vi "S4GUI.vi"() -> ()   [LabVIEW 2018] (continued)
                      frame #4 {
                        # "Gain"
                        n596 = Unbundle By Name(w1331) -> ("EM_GAIN"=w1330:u16)
                        n597 = Number To Decimal String(number=w1330) -> (decimal integer string=w1329:string)  [unwired: 1 in]
                      }
                      frame #5 {
                        # "Readout"
                        n598 = Unbundle By Name(w1335) -> ("EM_MODE"=w1334:u8, "READOUT_RATE"=w1333:u8)
                        n599 = case shown="0, Default" w1334 {
                          tunnel: w1333 -> [w1337 w1343]
                          tunnel: [w1336 w1342] -> w1332
                          frame 0, Default {
                            n600 = case shown="0, Default" w1337 {
                              tunnel: ["30 MHz" ("EmActive1") "20 MHz" ("EmActive1") "10 MHz" ("EmActive1") "1 MHz" ("EmActive1")] -> w1336
                              frame 0, Default {
                              }
                              frame 1 {
                              }
                              frame 2 {
                              }
                              frame 3 {
                              }
                            }
                          }
                          frame 1 {
                            n601 = case shown="1" w1343 {
                              tunnel: ["1 MHz" ("EmActive1") "0.1 MHz" ("EmActive1")] -> w1342
                              frame 0, Default {
                              }
                              frame 1 {
                              }
                            }
                          }
                        }
                      }
                    }
                  }
                }
                n602 = Unbundle By Name(w1220) -> ("INITIAL_LINE"=w1225:u16, "INITIAL_COLUMN"=w1223:u16, "FINAL_LINE"=w1226:u16, "FINAL_COLUMN"=w1224:u16, "VBIN"=w1229:u16, "HBIN"=w1285:u16, "PREAMP"=w1228:u8, "EM_GAIN"=w1227:u16, "READOUT_RATE"=w1222:u8, "SHUTTER_OPENNING_TIME"=w1284:u16, "SHUTTER_CLOSING_TIME"=w1283:u16, "VERTICAL_SHIFT_SPEED"=w1282:u8, "READ_MODE"=w1281:u8, "VERTICAL_CLOCK_VOLTAGE"=w1280:u8, "AD_CHANNEL"=w1279:u32, "SHUTTER_MODE"=w1274:u8, "SHUTTER_TTL"=w1275:u8, "TRIGGER_MODE"=w1276:u8, "FRAME_TRANSFER"=w1277:bool, "ACQUISITION_MODE"=w1278:u8, "EM_MODE"=w1221:u8)
                n603 = Not(x=w1248) -> (.not. x?=w1268:bool)
                n604 = Not(x=w1247) -> (.not. x?=w1266:bool)
                n605 = Not(x=w1246) -> (.not. x?=w1267:bool)
                n606 = Not(x=w1245) -> (.not. x?=w1265:bool)
                n607 = Not(x=w1251) -> (.not. x?=w1270:bool)
                n608 = Not(x=w1250) -> (.not. x?=w1269:bool)
                n609 = Not(x=w1249) -> (.not. x?=w1271:bool)
                n610 = property on="Image FInal Column 3" class="DigNum (strict)"("Blinking"=w1268) -> ()  [unwired: 2 in, 2 out]
                n611 = property on="Frame Transfer 3" class="Bool (strict)"("Blinking"=w1266) -> ()  [unwired: 2 in, 2 out]
                n612 = property on="Vertical Clock Voltage 3" class="Ring (strict)"("Blinking"=w1267) -> ()  [unwired: 2 in, 2 out]
                n613 = property on="A/D Channel 3" class="DigNum (strict)"("Blinking"=w1265) -> ()  [unwired: 2 in, 2 out]
                n614 = property on="Image Initial Line 3" class="DigNum (strict)"("Blinking"=w1270) -> ()  [unwired: 2 in, 2 out]
                n615 = property on="Image Initial Column 3" class="DigNum (strict)"("Blinking"=w1269) -> ()  [unwired: 2 in, 2 out]
                n616 = property on="Image Final Line 3" class="DigNum (strict)"("Blinking"=w1271) -> ()  [unwired: 2 in, 2 out]
                n617 = Not(x=w1240) -> (.not. x?=w1261:bool)
                n618 = Not(x=w1239) -> (.not. x?=w1263:bool)
                n619 = Not(x=w1238) -> (.not. x?=w1262:bool)
                n620 = Not(x=w1237) -> (.not. x?=w1264:bool)
                n621 = Not(x=w1244) -> (.not. x?=w1260:bool)
                n622 = Not(x=w1243) -> (.not. x?=w1242:bool)
                n623 = Not(x=w1241) -> (.not. x?=w1259:bool)
                n624 = property on="Shutter Openning Time 3" class="DigNum (strict)"("Blinking"=w1261) -> ()  [unwired: 2 in, 2 out]
                n625 = property on="Shutter Closing Time 3" class="DigNum (strict)"("Blinking"=w1263) -> ()  [unwired: 2 in, 2 out]
                n626 = property on="Vertical Binning 3" class="DigNum (strict)"("Blinking"=w1262) -> ()  [unwired: 2 in, 2 out]
                n627 = property on="Horizontal Binning 3" class="DigNum (strict)"("Blinking"=w1264) -> ()  [unwired: 2 in, 2 out]
                n628 = property on="CCD EM Gain 3" class="DigNum (strict)"("Blinking"=w1260) -> ()  [unwired: 2 in, 2 out]
                n629 = property on="Shutter Mode 3" class="Ring (strict)"("Blinking"=w1242) -> ()  [unwired: 2 in, 2 out]
                n630 = property on="Shutter TTL 3" class="Ring (strict)"("Blinking"=w1259) -> ()  [unwired: 2 in, 2 out]
                n631 = local read "Cameras Cluster"() -> (w1287:T6)
                n632 = Bundle By Name(cluster=w1287, "Current Configuration.Image Initial Line 3"=w1225, "Current Configuration.Image Initial Column 3"=w1223, "Current Configuration.Image Final Line 3"=w1226, "Current Configuration.Image FInal Column 3"=w1224, "Current Configuration.Vertical Binning 3"=w1229, "Current Configuration.Horizontal Binning 3"=w1285, "Current Configuration.Pre-amplification Gain 3"=w1228, "Current Configuration.CCD EM Gain 3"=w1227, "Current Configuration.Readout Rate 3"=w1222, "Current Configuration.Shutter Openning Time 3"=w1284, "Current Configuration.Shutter Closing Time 3"=w1283, "Current Configuration.Vertical Shift Speed 3"=w1282, "Current Configuration.Read Mode 3"=w1281, "Current Configuration.Vertical Clock Voltage 3"=w1280, "Current Configuration.A/D Channel 3"=w1279, "Current Configuration.Shutter Mode 3"=w1274, "Current Configuration.Shutter TTL 3"=w1275, "Current Configuration.Trigger Mode 3"=w1276, "Current Configuration.Frame Transfer 3"=w1277, "Current Configuration.Acquisition Mode 3"=w1278, "Current Configuration.CCD EM Mode 3"=w1221) -> (w1286:T6)
                n633 = Not(x=w1236) -> (.not. x?=w1252:bool)
                n634 = Not(x=w1232) -> (.not. x?=w1255:bool)
                n635 = Not(x=w1231) -> (.not. x?=w1253:bool)
                n636 = Not(x=w1230) -> (.not. x?=w1254:bool)
                n637 = Not(x=w1235) -> (.not. x?=w1257:bool)
                n638 = Not(x=w1234) -> (.not. x?=w1256:bool)
                n639 = Not(x=w1233) -> (.not. x?=w1258:bool)
                n640 = local write "RO3"(w1214) -> ()
                n641 = local write "B3"(w1216) -> ()
                n642 = local write "PA3"(w1217) -> ()
                n643 = local write "EA3"(w1218) -> ()
                n644 = local write "G3"(w1215) -> ()
                n645 = local write "SI3"(w1219) -> ()
                n646 = property on="Acquisition Mode 3" class="Ring (strict)"("Blinking"=w1252) -> ()  [unwired: 2 in, 2 out]
                n647 = property on="Readout Rate 3" class="Ring (strict)"("Blinking"=w1255) -> ()  [unwired: 2 in, 2 out]
                n648 = property on="Vertical Shift Speed 3" class="Ring (strict)"("Blinking"=w1253) -> ()  [unwired: 2 in, 2 out]
                n649 = property on="CCD EM Mode 3" class="Ring (strict)"("Blinking"=w1254) -> ()  [unwired: 2 in, 2 out]
                n650 = property on="Trigger Mode 3" class="Ring (strict)"("Blinking"=w1257) -> ()  [unwired: 2 in, 2 out]
                n651 = property on="Read Mode 3" class="Ring (strict)"("Blinking"=w1256) -> ()  [unwired: 2 in, 2 out]
                n652 = property on="Pre-amplification Gain 3" class="Ring (strict)"("Blinking"=w1258) -> ()  [unwired: 2 in, 2 out]
                n653 = local write "Cameras Cluster"(w1286) -> ()
                n654 = Compound Arithmetic op=AND(w1236, w1235, w1234, w1233, w1232, w1231, w1230, w1244, w1243, w1241, w1240, w1239, w1238, w1237, w1251, w1250, w1249, w1248, w1247, w1246, w1245) -> (→"CCD checked 3":bool)
              }
              frame #18 {
                # "Carrega coluna do Channel 4"
                # "Aba:  Eng->Camera"
                n655 = Unbundle By Name(w1421) -> ("ChannelD_CCD"=w1353:T21, "CHD_Checked Params"=w1406:T22, "ChannelD_Status.connection"=w1352:bool)
                n656 = Unbundle By Name(w1406) -> ("ACQUISITION_MODE"=w1370:bool, "TRIGGER_MODE"=w1369:bool, "READ_MODE"=w1368:bool, "PREAMP"=w1366:bool, "READOUT_RATE"=w1365:bool, "VERTICAL_SHIFT_SPEED"=w1364:bool, "EM_MODE"=w1363:bool, "EM_GAIN"=w1377:bool, "SHUTTER_MODE"=w1376:bool, "SHUTTER_TTL"=w1375:bool, "SHUTTER_OPENING_TIME"=w1374:bool, "SHUTTER_CLOSING_TIME"=w1373:bool, "VBIN"=w1372:bool, "HBIN"=w1371:bool, "INITIAL_LINE"=w1384:bool, "INITIAL_COLUMN"=w1383:bool, "FINAL_LINE"=w1382:bool, "FINAL_COLUMN"=w1381:bool, "FRAME_TRANSFER"=w1380:bool, "VERTICAL_CLOCK_VOLTAGE"=w1379:bool, "AD_CHANNEL"=w1378:bool)
                n657 = case shown="False" w1352 {
                  tunnel: w1353 -> [_ w1429]
                  tunnel: [w1422 w1428] -> w1351
                  tunnel: [w1422 w1427] -> w1350
                  tunnel: [w1422 w1426] -> w1349
                  tunnel: [w1422 w1425] -> w1348
                  tunnel: [w1422 w1424] -> w1347
                  tunnel: [w1422 w1423] -> w1346
                  frame False {
                    w1422 = ""
                  }
                  frame True {
                    n658 = stacked-sequence "Atualizacao dos indicadores inferiores do CANAL D da tela principal" {
                      tunnel: w1429 -> [w1444 w1447 w1452 w1461 w1464 w1468]
                      tunnel: [w1430 _ _ _ _ _] -> w1428
                      tunnel: [_ w1445 _ _ _ _] -> w1427
                      tunnel: [_ _ w1450 _ _ _] -> w1426
                      tunnel: [_ _ _ w1455 _ _] -> w1425
                      tunnel: [_ _ _ _ w1462 _] -> w1424
                      tunnel: [_ _ _ _ _ w1465] -> w1423
                      frame #0 {
                        # "SubImage"
                        n659 = Unbundle By Name(w1444) -> ("INITIAL_LINE"=w1442:u16, "FINAL_LINE"=w1441:u16, "INITIAL_COLUMN"=w1440:u16, "FINAL_COLUMN"=w1439:u16)
                        n660 = Number To Decimal String(number=w1442) -> (decimal integer string=w1438:string)  [unwired: 1 in]
                        n661 = Number To Decimal String(number=w1441) -> (decimal integer string=w1436:string)  [unwired: 1 in]
                        n662 = Number To Decimal String(number=w1440) -> (decimal integer string=w1434:string)  [unwired: 1 in]
                        n663 = Number To Decimal String(number=w1439) -> (decimal integer string=w1432:string)  [unwired: 1 in]
                        n664 = Concatenate Strings("[", w1438, ":", w1436, ",", w1434, ":", w1432, "]") -> (w1430:string)
                      }
                      frame #1 {
                        # "Em Active"
                        n665 = Unbundle By Name(w1447) -> ("EM_MODE"=w1446:u8)
                        n666 = case shown="0, Default" w1446 {
                          tunnel: ["Electron M." ("EmActive1") "Convent." ("EmActive1")] -> w1445
                          frame 0, Default {
                          }
                          frame 1 {
                          }
                        }
                      }
                      frame #2 {
                        # "Pre Amp"
                        n667 = Unbundle By Name(w1452) -> ("PREAMP"=w1451:u8)
                        n668 = case shown="1" w1451 {
                          tunnel: ["Gain 1" ("EmActive1") "Gain 2" ("EmActive1")] -> w1450
                          frame 0, Default {
                          }
                          frame 1 {
                          }
                        }
                      }
                      frame #3 {
                        # "Binning"
                        n669 = Unbundle By Name(w1461) -> ("VBIN"=w1460:u16, "HBIN"=w1459:u16)
                        n670 = Number To Decimal String(number=w1459) -> (decimal integer string=w1456:string)  [unwired: 1 in]
                        n671 = Number To Decimal String(number=w1460) -> (decimal integer string=w1458:string)  [unwired: 1 in]
                        n672 = Concatenate Strings(w1458, "x", w1456) -> (w1455:string)
                      }
                      frame #4 {
                        # "Gain"
                        n673 = Unbundle By Name(w1464) -> ("EM_GAIN"=w1463:u16)
                        n674 = Number To Decimal String(number=w1463) -> (decimal integer string=w1462:string)  [unwired: 1 in]
                      }
                      frame #5 {
                        # "Readout"
                        n675 = Unbundle By Name(w1468) -> ("EM_MODE"=w1467:u8, "READOUT_RATE"=w1466:u8)
                        n676 = case shown="0, Default" w1467 {
                          tunnel: w1466 -> [w1470 w1476]
                          tunnel: [w1469 w1475] -> w1465
                          frame 0, Default {
                            n677 = case shown="0, Default" w1470 {
                              tunnel: ["30 MHz" ("EmActive1") "20 MHz" ("EmActive1") "10 MHz" ("EmActive1") "1 MHz" ("EmActive1")] -> w1469
                              frame 0, Default {
                              }
                              frame 1 {
                              }
                              frame 2 {
                              }
                              frame 3 {
                              }
                            }
                          }
                          frame 1 {
                            n678 = case shown="1" w1476 {
                              tunnel: ["1 MHz" ("EmActive1") "0.1 MHz" ("EmActive1")] -> w1475
                              frame 0, Default {
                              }
                              frame 1 {
                              }
                            }
                          }
                        }
                      }
                    }
                  }
                }
                n679 = Unbundle By Name(w1353) -> ("INITIAL_LINE"=w1358:u16, "INITIAL_COLUMN"=w1356:u16, "FINAL_LINE"=w1359:u16, "FINAL_COLUMN"=w1357:u16, "VBIN"=w1362:u16, "HBIN"=w1418:u16, "PREAMP"=w1361:u8, "EM_GAIN"=w1360:u16, "READOUT_RATE"=w1355:u8, "SHUTTER_OPENNING_TIME"=w1417:u16, "SHUTTER_CLOSING_TIME"=w1416:u16, "VERTICAL_SHIFT_SPEED"=w1415:u8, "READ_MODE"=w1414:u8, "VERTICAL_CLOCK_VOLTAGE"=w1413:u8, "AD_CHANNEL"=w1412:u32, "SHUTTER_MODE"=w1407:u8, "SHUTTER_TTL"=w1408:u8, "TRIGGER_MODE"=w1409:u8, "FRAME_TRANSFER"=w1410:bool, "ACQUISITION_MODE"=w1411:u8, "EM_MODE"=w1354:u8)
                n680 = Not(x=w1381) -> (.not. x?=w1401:bool)
                n681 = Not(x=w1380) -> (.not. x?=w1399:bool)
                n682 = Not(x=w1379) -> (.not. x?=w1400:bool)
                n683 = Not(x=w1378) -> (.not. x?=w1398:bool)
                n684 = Not(x=w1384) -> (.not. x?=w1403:bool)
                n685 = Not(x=w1383) -> (.not. x?=w1402:bool)
                n686 = Not(x=w1382) -> (.not. x?=w1404:bool)
                n687 = property on="Image FInal Column 4" class="DigNum (strict)"("Blinking"=w1401) -> ()  [unwired: 2 in, 2 out]
                n688 = property on="Frame Transfer 4" class="Bool (strict)"("Blinking"=w1399) -> ()  [unwired: 2 in, 2 out]
                n689 = property on="Vertical Clock Voltage 4" class="Ring (strict)"("Blinking"=w1400) -> ()  [unwired: 2 in, 2 out]
                n690 = property on="A/D Channel 4" class="DigNum (strict)"("Blinking"=w1398) -> ()  [unwired: 2 in, 2 out]
                n691 = property on="Image Initial Line 4" class="DigNum (strict)"("Blinking"=w1403) -> ()  [unwired: 2 in, 2 out]
                n692 = property on="Image Initial Column 4" class="DigNum (strict)"("Blinking"=w1402) -> ()  [unwired: 2 in, 2 out]
                n693 = property on="Image Final Line 4" class="DigNum (strict)"("Blinking"=w1404) -> ()  [unwired: 2 in, 2 out]
                n694 = Not(x=w1374) -> (.not. x?=w1394:bool)
                n695 = Not(x=w1373) -> (.not. x?=w1396:bool)
                n696 = Not(x=w1372) -> (.not. x?=w1395:bool)
                n697 = Not(x=w1371) -> (.not. x?=w1397:bool)
                n698 = Not(x=w1377) -> (.not. x?=w1392:bool)
                n699 = Not(x=w1376) -> (.not. x?=w1393:bool)
                n700 = Not(x=w1375) -> (.not. x?=w1391:bool)
                n701 = property on="Shutter Openning Time 4" class="DigNum (strict)"("Blinking"=w1394) -> ()  [unwired: 2 in, 2 out]
                n702 = property on="Shutter Closing Time 4" class="DigNum (strict)"("Blinking"=w1396) -> ()  [unwired: 2 in, 2 out]
                n703 = property on="Vertical Binning 4" class="DigNum (strict)"("Blinking"=w1395) -> ()  [unwired: 2 in, 2 out]
                n704 = property on="Horizontal Binning 4" class="DigNum (strict)"("Blinking"=w1397) -> ()  [unwired: 2 in, 2 out]
                n705 = property on="CCD EM Gain 4" class="DigNum (strict)"("Blinking"=w1392) -> ()  [unwired: 2 in, 2 out]
                n706 = property on="Shutter Mode 4" class="Ring (strict)"("Blinking"=w1393) -> ()  [unwired: 2 in, 2 out]
                n707 = property on="Shutter TTL 4" class="Ring (strict)"("Blinking"=w1391) -> ()  [unwired: 2 in, 2 out]
                n708 = local read "Cameras Cluster"() -> (w1420:T6)
                n709 = Bundle By Name(cluster=w1420, "Current Configuration.Image Initial Line 4"=w1358, "Current Configuration.Image Initial Column 4"=w1356, "Current Configuration.Image Final Line 4"=w1359, "Current Configuration.Image FInal Column 4"=w1357, "Current Configuration.Vertical Binning 4"=w1362, "Current Configuration.Horizontal Binning 4"=w1418, "Current Configuration.Pre-amplification Gain 4"=w1361, "Current Configuration.CCD EM Gain 4"=w1360, "Current Configuration.Readout Rate 4"=w1355, "Current Configuration.Shutter Openning Time 4"=w1417, "Current Configuration.Shutter Closing Time 4"=w1416, "Current Configuration.Vertical Shift Speed 4"=w1415, "Current Configuration.Read Mode 4"=w1414, "Current Configuration.Vertical Clock Voltage 4"=w1413, "Current Configuration.A/D Channel 4"=w1412, "Current Configuration.Shutter Mode 4"=w1407, "Current Configuration.Shutter TTL 4"=w1408, "Current Configuration.Trigger Mode 4"=w1409, "Current Configuration.Frame Transfer 4"=w1410, "Current Configuration.Acquisition Mode 4"=w1411, "Current Configuration.CCD EM Mode 4"=w1354) -> (w1419:T6)
                n710 = local write "SI4"(w1351) -> ()
                n711 = local write "RO4"(w1346) -> ()
                n712 = local write "PA4"(w1349) -> ()
                n713 = local write "EA4"(w1350) -> ()
                n714 = local write "G4"(w1347) -> ()
                n715 = local write "B4"(w1348) -> ()
                n716 = Not(x=w1370) -> (.not. x?=w1385:bool)
                n717 = Not(x=w1365) -> (.not. x?=w1388:bool)
                n718 = Not(x=w1364) -> (.not. x?=w1386:bool)
                n719 = Not(x=w1363) -> (.not. x?=w1387:bool)
                n720 = Not(x=w1369) -> (.not. x?=w1389:bool)
                n721 = Not(x=w1368) -> (.not. x?=w1367:bool)
                n722 = Not(x=w1366) -> (.not. x?=w1390:bool)
                n723 = property on="Acquisition Mode 4" class="Ring (strict)"("Blinking"=w1385) -> ()  [unwired: 2 in, 2 out]
                n724 = property on="Readout Rate 4" class="Ring (strict)"("Blinking"=w1388) -> ()  [unwired: 2 in, 2 out]
                n725 = property on="Vertical Shift Speed 4" class="Ring (strict)"("Blinking"=w1386) -> ()  [unwired: 2 in, 2 out]
                n726 = property on="CCD EM Mode 4" class="Ring (strict)"("Blinking"=w1387) -> ()  [unwired: 2 in, 2 out]
                n727 = property on="Trigger Mode 4" class="Ring (strict)"("Blinking"=w1389) -> ()  [unwired: 2 in, 2 out]
                n728 = property on="Read Mode 4" class="Ring (strict)"("Blinking"=w1367) -> ()  [unwired: 2 in, 2 out]
                n729 = property on="Pre-amplification Gain 4" class="Ring (strict)"("Blinking"=w1390) -> ()  [unwired: 2 in, 2 out]
                n730 = local write "Cameras Cluster"(w1419) -> ()
                n731 = Compound Arithmetic op=AND(w1370, w1369, w1368, w1366, w1365, w1364, w1363, w1377, w1376, w1375, w1374, w1373, w1372, w1371, w1384, w1383, w1382, w1381, w1380, w1379, w1378) -> (→"CCD checked 4":bool)
              }
            }
            n732 = stacked-sequence {
              tunnel: w172 -> [w186 w190 w198 w205 w219]
              tunnel: w171 -> [w185 w189 w197 w204 w218]
              tunnel: [_ _ _ _ w210] -> w163
              tunnel: [_ _ _ _ w211] -> w162
              frame #0 {
                n733 = call-dynamic "Read AcquisitionA.vi"("error in (no error)"=w185, "S4ACS_GUI in"=w186) -> ("error out"=w182:errorcluster, "Acquisition.lvclass"=w184:refnum<class "Acquisition.lvclass">)  [unwired: 7 in, 1 out]
                n734 = call-dynamic "Read Channel.vi"("error in (no error)"=w182, "Acquisition in"=w184) -> ("error out"=w181:errorcluster, "Channel.lvclass"=w183:refnum<class "Channel.lvclass">)  [unwired: 7 in, 1 out]
                n735 = call-dynamic "Read CyclesDone.vi"("error in (no error)"=w181, "Channel in"=w183) -> ("error out"=→"error out 6":errorcluster, "CyclesDone"=→"Cycles Done ch1":u32)  [unwired: 7 in, 1 out]
              }
              frame #1 {
                n736 = call "Read AcquisitionB.vi"("error in (no error)"=w189, "S4ACS_GUI in"=w190) -> ("error out"=w192:errorcluster, "Acquisition.lvclass"=w193:refnum<class "Acquisition.lvclass">)  [unwired: 7 in, 1 out]
                n737 = call-dynamic "Read Channel.vi"("error in (no error)"=w192, "Acquisition in"=w193) -> ("error out"=w191:errorcluster, "Channel.lvclass"=w194:refnum<class "Channel.lvclass">)  [unwired: 7 in, 1 out]
                n738 = call-dynamic "Read CyclesDone.vi"("error in (no error)"=w191, "Channel in"=w194) -> ("error out"=→"error out 4":errorcluster, "CyclesDone"=→"Cycles Done ch2":u32)  [unwired: 7 in, 1 out]
              }
              frame #2 {
                n739 = call-dynamic "Read AcquisitionC.vi"("error in (no error)"=w197, "S4ACS_GUI in"=w198) -> ("error out"=w200:errorcluster, "Acquisition.lvclass"=w201:refnum<class "Acquisition.lvclass">)  [unwired: 7 in, 1 out]
                n740 = call-dynamic "Read Channel.vi"("error in (no error)"=w200, "Acquisition in"=w201) -> ("error out"=w199:errorcluster, "Channel.lvclass"=w202:refnum<class "Channel.lvclass">)  [unwired: 7 in, 1 out]
                n741 = call-dynamic "Read CyclesDone.vi"("error in (no error)"=w199, "Channel in"=w202) -> ("error out"=→"error out 5":errorcluster, "CyclesDone"=→"Cycles Done ch3":u32)  [unwired: 7 in, 1 out]
              }
              frame #3 {
                n742 = call-dynamic "Read AcquisitionD.vi"("error in (no error)"=w204, "S4ACS_GUI in"=w205) -> ("error out"=w207:errorcluster, "Acquisition.lvclass"=w208:refnum<class "Acquisition.lvclass">)  [unwired: 7 in, 1 out]
                n743 = call-dynamic "Read Channel.vi"("error in (no error)"=w207, "Acquisition in"=w208) -> ("error out"=w206:errorcluster, "Channel.lvclass"=w209:refnum<class "Channel.lvclass">)  [unwired: 7 in, 1 out]
                n744 = call-dynamic "Read CyclesDone.vi"("error in (no error)"=w206, "Channel in"=w209) -> ("CyclesDone"=→"Cycles Done ch4":u32)  [unwired: 7 in, 2 out]
              }
              frame #4 {
                (unwired) cluster{"AG status":bool, "rotator":dbl} {"AG status"=FALSE, "rotator"=0.0} ("element")
                n745 = call-dynamic "Read guider queue.vi"("error in (no error)"=w218, "S4GUI in"=w219) -> ("error out"=w213:errorcluster, "guider queue"=w217:refnum<queue>, "S4GUI out"=w212:refnum<class "S4GUI.lvclass">)  [unwired: 7 in]
                n746 = Get Queue Status(queue=w217, error in (no error)=w213) -> (queue out=w215:refnum<queue>, error out=w214:errorcluster, # elements in queue=w216:i32)  [unwired: 1 in, 5 out]
                n747 = case shown="Default" w216 {
                  tunnel: w215 -> [_ w232]
                  tunnel: w214 -> [w220 w231]
                  tunnel: w212 -> [w221 w226]
                  tunnel: [w220 w224] -> w211
                  tunnel: [w221 w225] -> w210
                  frame 0 {
                  }
                  frame Default {
                    n748 = Dequeue Element(queue=w232, error in (no error)=w231) -> (queue out=w229:refnum<queue>, element=w228:cluster{"AG status":bool, "rotator":dbl}, error out=w230:errorcluster)  [unwired: 1 in, 1 out]
                    n749 = Unbundle By Name(w228) -> ("AG status"=→"GUIDER":bool, "rotator"=w222:dbl)
                    "rotator" <- w222
                    n750 = Flush Queue(queue=w229, error in (no error)=w230) -> (error out=w223:errorcluster)  [unwired: 2 out]
                    n751 = call-dynamic "Write rotator.vi"("error in (no error)"=w223, "rotator"=w222, "S4GUI in"=w226) -> ("error out"=w224:errorcluster, "S4GUI out"=w225:refnum<class "S4GUI.lvclass">)  [unwired: 7 in]
                  }
                }
              }
            }
            n752 = call-dynamic "Read Obs_state.vi"("error in (no error)"=w162, "S4ACS_GUI in"=w163) -> ("error out"=w158:errorcluster, "Obs_state"=w159:u32, "S4ACS_GUI out"=w157:refnum<class "S4GUI.lvclass">)  [unwired: 7 in]
            n753 = In Range and Coerce(upper limit=u32 226, x=w159, lower limit=u32 220 ("upper limit")) -> (In Range?=w155:bool)  [unwired: 1 out]
            n754 = Select(t="STOP", s=w155, f="INIT") -> (s? t:f=w154:string)
            n755 = property on="Init mode" class="Bool"(error in=w158, "Blinking"=w155, "Caption.Visible"=w155, "BoolText.Text"=w154) -> (error out=w156:errorcluster)  [unwired: 1 in, 1 out]
            n756 = call-dynamic "Read cyclesDone.vi"("error in (no error)"=w156, "S4GUI in"=w157) -> ("error out"=w174:errorcluster, "cyclesDone"=→"#Cycles Done":u32, "S4GUI out"=w173:refnum<class "S4GUI.lvclass">)  [unwired: 7 in]
            n757 = call "Read Instrument.lvclass.vi"("error in (no error)"=w174, "S4ACS_GUI in"=w173) -> ("error out"=w168:errorcluster, "Instrument.lvclass"=w165:refnum<class "Instrument.lvclass">, "S4ACS_GUI out"=w170:refnum<class "S4GUI.lvclass">)  [unwired: 7 in]
            n758 = call-dynamic "Write mode.vi"("error in (no error)"=w168, "mode"=w150, "Instrument in"=w165) -> ("error out"=w167:errorcluster, "Instrument out"=w164:refnum<class "Instrument.lvclass">)  [unwired: 7 in]
            n759 = call "Write Instrument.lvclass.vi"("error in (no error)"=w167, "Instrument.lvclass"=w164, "S4ACS_GUI in"=w170) -> ("error out"=w166:errorcluster, "S4ACS_GUI out"=w169:refnum<class "S4GUI.lvclass">)  [unwired: 7 in]
          }
        }
        n760 = Or(x="stop", y="stop 2") -> (x .or. y?=w133:bool)
      }
      event "Set from Input ch1": Value Change {
        # "ACS"
        # "GUI"
        # "EM_MODE = E.M."
        # "Readou Rate:\n30         0\n20         1     \n10         2\n1           3"
        # "EM_MODE = Conv"
        # "Readou Rate:\n1         0\n0.1      1"
        # "Readou Rate:\n1         0\n0.1      1     \n10       2\n20       3\n30       4"
        n761 = event-data() -> ()  [unwired: 1 in, 6 out]
        n762 = local read "Input Cluster"() -> (w1489:T5)
        n763 = Unbundle By Name(w1489) -> ("Parameters"=w1488:T23)
        n764 = Unbundle By Name(w1488) -> ("Image \nInitial Line"=w1517:u16, "Image\nInitial Column"=w1516:u16, "Image\nFinal Line"=w1515:u16, "Image\nFInal Column"=w1514:u16, "Vertical\nBinning"=w1513:u16, "Horizontal\nBinning"=w1512:u16, "Pre-amplification\nGain"=w1511:u8, "CCD\nEM Gain"=w1510:u16, "Readout\nRate"=w1509:u8, "Shutter\nOpenning Time"=w1508:i32, "Shutter\nClosing Time"=w1507:i32, "Vertical\nShift Speed"=w1506:u8, "Read\nMode"=w1505:u8, "Vertical\nClock Voltage"=w1504:u8, "A/D \nChannel"=w1503:u32, "Shutter\nMode"=w1502:u16, "Shutter\nTTL"=w1501:u16, "Trigger\nMode"=w1500:u16, "Frame\nTransfer"=w1499:bool, "Acquisition\nMode"=w1498:u8, "CCD \nEM Mode"=w1497:u8)
        n765 = call-dynamic "Read AcquisitionA.vi"("error in (no error)"=w1480, "S4ACS_GUI in"=w1481) -> ("error out"=w1540:errorcluster, "Acquisition.lvclass"=w1544:refnum<class "Acquisition.lvclass">, "S4ACS_GUI out"=w1545:refnum<class "S4GUI.lvclass">)  [unwired: 7 in]
        n766 = call-dynamic "Read Channel.vi"("error in (no error)"=w1540, "Acquisition in"=w1544) -> ("error out"=w1539:errorcluster, "Channel.lvclass"=w1542:refnum<class "Channel.lvclass">, "Acquisition out"=w1543:refnum<class "Acquisition.lvclass">)  [unwired: 7 in]
        n767 = call-dynamic "Read Interface.vi"("error in (no error)"=w1539, "Channel in"=w1542) -> ("error out"=w1521:errorcluster, "Interface.lvclass"=w1522:refnum<class "Interface.lvclass">, "Channel out"=w1541:refnum<class "Channel.lvclass">)  [unwired: 7 in]
        n768 = call-dynamic "Get CCD_Config.vi"("error in (no error)"=w1521, "Interface in"=w1522) -> ("error out"=w1518:errorcluster, "output cluster"=w1520:T24, "Interface out"=w1519:refnum<class "Interface.lvclass">)  [unwired: 7 in]
        n769 = Bundle By Name(cluster=w1520, "INITIAL_LINE"=w1517, "INITIAL_COLUMN"=w1516, "FINAL_LINE"=w1515, "FINAL_COLUMN"=w1514, "VBIN"=w1513, "HBIN"=w1512, "PREAMP"=w1511, "EM_GAIN"=w1510, "READOUT_RATE"=w1509, "SHUTTER_OPENING_TIME"=w1508, "SHUTTER_CLOSING_TIME"=w1507, "VERTICAL_SHIFT_SPEED"=w1506, "READ_MODE"=w1505, "VERTICAL_CLOCK_VOLTAGE"=w1504, "AD_CHANNEL"=w1503, "SHUTTER_MODE"=w1502, "SHUTTER_TTL"=w1501, "TRIGGER_MODE"=w1500, "FRAME_TRANSFER"=w1499, "ACQUISITION_MODE"=w1498, "EM_MODE"=w1497) -> (w1487:T24)
        n770 = call-dynamic "Set CCD_Config.vi"("error in (no error)"=w1518, "input cluster"=w1487, "Interface in"=w1519) -> ("error out"=w1525:errorcluster, "Interface out"=w1526:refnum<class "Interface.lvclass">)  [unwired: 7 in]
        n771 = Flatten To String(anything=w1487, error in (no error)=w1525) -> (data string=w1528:string, error out=w1527:errorcluster)  [unwired: 2 in, 1 out]
        n772 = call "Write flatted cluster.vi"("error in (no error)"=w1527, "flatted cluster"=w1528, "Interface in"=w1526) -> ("error out"=w1524:errorcluster, "Interface out"=w1523:refnum<class "Interface.lvclass">)  [unwired: 7 in]
        n773 = call-dynamic "Write Interface.vi"("error in (no error)"=w1524, "Interface.lvclass"=w1523, "Channel in"=w1541) -> ("error out"=w1492:errorcluster, "Channel out"=w1495:refnum<class "Channel.lvclass">)  [unwired: 7 in]
        n774 = call "Write section_name.vi"("error in (no error)"=w1492, "section_name"="CCD_ACS1", "Channel in"=w1495) -> ("error out"=w1491:errorcluster, "Channel out"=w1494:refnum<class "Channel.lvclass">)  [unwired: 7 in]
        n775 = call-dynamic "save config.vi"("error in (no error)"=w1491, "file config"="lastsaved.cfg", "Channel in"=w1494) -> ("error out"=w1490:errorcluster, "Channel out"=w1493:refnum<class "Channel.lvclass">)  [unwired: 7 in]
        n776 = call-dynamic "Read State Machine.vi"("error in (no error)"=w1490, "Device in"=w1493) -> ("error out"=w1535:errorcluster, "State Machine.lvclass"=w1537:refnum<class "State Machine.lvclass">, "Device out"=w1538:refnum<class "Channel.lvclass">)  [unwired: 7 in]
        n777 = call-dynamic "Write State.vi"("error in (no error)"=w1535, "State"=60, "State Machine in"=w1537) -> ("error out"=w1534:errorcluster, "State Machine out"=w1536:refnum<class "State Machine.lvclass">)  [unwired: 7 in]
        n778 = call-dynamic "Write State Machine.vi"("error in (no error)"=w1534, "State Machine.lvclass"=w1536, "Device in"=w1538) -> ("error out"=w1531:errorcluster, "Device out"=w1532:refnum<class "Channel.lvclass">)  [unwired: 7 in]
        n779 = call-dynamic "Write Channel.vi"("error in (no error)"=w1531, "Channel.lvclass"=w1532, "Acquisition in"=w1543) -> ("error out"=w1530:errorcluster, "Acquisition out"=w1529:refnum<class "Acquisition.lvclass">)  [unwired: 7 in]
        n780 = call-dynamic "Write AcquisitionA.vi"("error in (no error)"=w1530, "Acquisition.lvclass"=w1529, "S4ACS_GUI in"=w1545) -> ("error out"=w1482:errorcluster, "S4ACS_GUI out"=w1483:refnum<class "S4GUI.lvclass">)  [unwired: 7 in]
        n781 = call "Write cfg file.vi"("error in (no error)"=w1482, "cfg file"="lastsaved.cfg", "S4ACS_GUI in"=w1483) -> ("error out"=w1485:errorcluster, "S4ACS_GUI out"=w1486:refnum<class "S4GUI.lvclass">)  [unwired: 7 in]
      }
      event "Input Cluster.Parameters.CCD \nEM Mode": Value Change {
        n782 = event-data() -> ()  [unwired: 1 in, 6 out]
        n783 = local read "Input Cluster"() -> (w1560:T5)
        n784 = Unbundle By Name(w1560) -> ("Parameters"=w1561:T23)
        n785 = Unbundle By Name(w1561) -> ("Readout\nRate"=→"Readout\nRate":u8, "CCD \nEM Mode"=w1555:u8)
        n786 = case shown="1" w1555 {
          tunnel: [string[] ["30 MHz", "20 MHz", "10 MHz", "1 MHz"] ("Strings []") string[] ["1 MHz", "0.1 MHz"] ("Strings []")] -> w1554
          tunnel: [u8 3 u8 0] -> w1553
          frame 0, Default {
          }
          frame 1 {
          }
        }
        n787 = local read "Cameras Cluster"() -> (w1548:T6)
        n788 = Unbundle By Name(w1548) -> ("Current Configuration"=w1549:T25)
        n789 = flat-sequence {
          tunnel: w1553 -> [w1563]
          tunnel: w1554 -> [w1562]
          tunnel: w1555 -> [w1564]
          tunnel: [w1564] -> w1552
          tunnel: [w1563] -> w1550
          tunnel: w1561 -> [w1570]
          tunnel: [w1569] -> w1559
          tunnel: w1552 -> [w1565]
          tunnel: w1550 -> [w1566]
          tunnel: w1549 -> [w1568]
          tunnel: [w1567] -> w1547
          frame #0 {
            n790 = property on="Readout\nRate" class="Ring (strict)"("Strings []"=w1562) -> ()  [unwired: 2 in, 2 out]
            n791 = property on="Readout Rate" class="Ring (strict)"("Strings []"=w1562) -> ()  [unwired: 2 in, 2 out]
            n792 = property on="Readout Rate 4" class="Ring (strict)"("Strings []"=w1562) -> ()  [unwired: 2 in, 2 out]
            n793 = property on="Readout Rate 2" class="Ring (strict)"("Strings []"=w1562) -> ()  [unwired: 2 in, 2 out]
            n794 = property on="Readout Rate 3" class="Ring (strict)"("Strings []"=w1562) -> ()  [unwired: 2 in, 2 out]
          }
          frame #1 {
            n795 = Bundle By Name(cluster=w1568, "Readout Rate"=w1566, "Read Mode"=w1565) -> (w1567:T25)
            n796 = Bundle By Name(cluster=w1570, "Readout\nRate"=w1566, "CCD \nEM Mode"=w1565) -> (w1569:T23)
          }
        }
        n797 = Bundle By Name(cluster=w1560, "Parameters"=w1559) -> (w1558:T5)
        n798 = Bundle By Name(cluster=w1548, "Current Configuration"=w1547) -> (w1546:T6)
        n799 = local write "Input Cluster"(w1558) -> ()
        n800 = local write "Cameras Cluster"(w1546) -> ()
      }
      event "Set from Input ch2": Value Change {
        n801 = event-data() -> ()  [unwired: 1 in, 6 out]
        n802 = local read "Input Cluster"() -> (w1583:T5)
        n803 = Unbundle By Name(w1583) -> ("Parameters"=w1582:T23)
        n804 = Unbundle By Name(w1582) -> ("Image \nInitial Line"=w1611:u16, "Image\nInitial Column"=w1610:u16, "Image\nFinal Line"=w1609:u16, "Image\nFInal Column"=w1608:u16, "Vertical\nBinning"=w1607:u16, "Horizontal\nBinning"=w1606:u16, "Pre-amplification\nGain"=w1605:u8, "CCD\nEM Gain"=w1604:u16, "Readout\nRate"=w1603:u8, "Shutter\nOpenning Time"=w1602:i32, "Shutter\nClosing Time"=w1601:i32, "Vertical\nShift Speed"=w1600:u8, "Read\nMode"=w1599:u8, "Vertical\nClock Voltage"=w1598:u8, "A/D \nChannel"=w1597:u32, "Shutter\nMode"=w1596:u16, "Shutter\nTTL"=w1595:u16, "Trigger\nMode"=w1594:u16, "Frame\nTransfer"=w1593:bool, "Acquisition\nMode"=w1592:u8, "CCD \nEM Mode"=w1591:u8)
        n805 = call "Read AcquisitionB.vi"("error in (no error)"=w1640, "S4ACS_GUI in"=w1641) -> ("error out"=w1634:errorcluster, "Acquisition.lvclass"=w1638:refnum<class "Acquisition.lvclass">, "S4ACS_GUI out"=w1639:refnum<class "S4GUI.lvclass">)  [unwired: 7 in]
        n806 = call-dynamic "Read Channel.vi"("error in (no error)"=w1634, "Acquisition in"=w1638) -> ("error out"=w1633:errorcluster, "Channel.lvclass"=w1636:refnum<class "Channel.lvclass">, "Acquisition out"=w1637:refnum<class "Acquisition.lvclass">)  [unwired: 7 in]
        n807 = call-dynamic "Read Interface.vi"("error in (no error)"=w1633, "Channel in"=w1636) -> ("error out"=w1615:errorcluster, "Interface.lvclass"=w1616:refnum<class "Interface.lvclass">, "Channel out"=w1635:refnum<class "Channel.lvclass">)  [unwired: 7 in]
        n808 = call-dynamic "Get CCD_Config.vi"("error in (no error)"=w1615, "Interface in"=w1616) -> ("error out"=w1612:errorcluster, "output cluster"=w1614:T24, "Interface out"=w1613:refnum<class "Interface.lvclass">)  [unwired: 7 in]
        n809 = Bundle By Name(cluster=w1614, "INITIAL_LINE"=w1611, "INITIAL_COLUMN"=w1610, "FINAL_LINE"=w1609, "FINAL_COLUMN"=w1608, "VBIN"=w1607, "HBIN"=w1606, "PREAMP"=w1605, "EM_GAIN"=w1604, "READOUT_RATE"=w1603, "SHUTTER_OPENING_TIME"=w1602, "SHUTTER_CLOSING_TIME"=w1601, "VERTICAL_SHIFT_SPEED"=w1600, "READ_MODE"=w1599, "VERTICAL_CLOCK_VOLTAGE"=w1598, "AD_CHANNEL"=w1597, "SHUTTER_MODE"=w1596, "SHUTTER_TTL"=w1595, "TRIGGER_MODE"=w1594, "FRAME_TRANSFER"=w1593, "ACQUISITION_MODE"=w1592, "EM_MODE"=w1591) -> (w1581:T24)
        n810 = call-dynamic "Set CCD_Config.vi"("error in (no error)"=w1612, "input cluster"=w1581, "Interface in"=w1613) -> ("error out"=w1619:errorcluster, "Interface out"=w1620:refnum<class "Interface.lvclass">)  [unwired: 7 in]
        n811 = Flatten To String(anything=w1581, error in (no error)=w1619) -> (data string=w1622:string, error out=w1621:errorcluster)  [unwired: 2 in, 1 out]
        n812 = call "Write flatted cluster.vi"("error in (no error)"=w1621, "flatted cluster"=w1622, "Interface in"=w1620) -> ("error out"=w1618:errorcluster, "Interface out"=w1617:refnum<class "Interface.lvclass">)  [unwired: 7 in]
        n813 = call-dynamic "Write Interface.vi"("error in (no error)"=w1618, "Interface.lvclass"=w1617, "Channel in"=w1635) -> ("error out"=w1586:errorcluster, "Channel out"=w1589:refnum<class "Channel.lvclass">)  [unwired: 7 in]
        n814 = call "Write section_name.vi"("error in (no error)"=w1586, "section_name"="CCD_ACS2", "Channel in"=w1589) -> ("error out"=w1585:errorcluster, "Channel out"=w1588:refnum<class "Channel.lvclass">)  [unwired: 7 in]
        n815 = call-dynamic "save config.vi"("error in (no error)"=w1585, "file config"="lastsaved.cfg", "Channel in"=w1588) -> ("error out"=w1584:errorcluster, "Channel out"=w1587:refnum<class "Channel.lvclass">)  [unwired: 7 in]
        n816 = call-dynamic "Read State Machine.vi"("error in (no error)"=w1584, "Device in"=w1587) -> ("error out"=w1629:errorcluster, "State Machine.lvclass"=w1631:refnum<class "State Machine.lvclass">, "Device out"=w1632:refnum<class "Channel.lvclass">)  [unwired: 7 in]
        n817 = call-dynamic "Write State.vi"("error in (no error)"=w1629, "State"=60, "State Machine in"=w1631) -> ("error out"=w1628:errorcluster, "State Machine out"=w1630:refnum<class "State Machine.lvclass">)  [unwired: 7 in]
        n818 = call-dynamic "Write State Machine.vi"("error in (no error)"=w1628, "State Machine.lvclass"=w1630, "Device in"=w1632) -> ("error out"=w1625:errorcluster, "Device out"=w1626:refnum<class "Channel.lvclass">)  [unwired: 7 in]
        n819 = call-dynamic "Write Channel.vi"("error in (no error)"=w1625, "Channel.lvclass"=w1626, "Acquisition in"=w1637) -> ("error out"=w1624:errorcluster, "Acquisition out"=w1623:refnum<class "Acquisition.lvclass">)  [unwired: 7 in]
        n820 = call "Write AcquisitionB.vi"("error in (no error)"=w1624, "Acquisition.lvclass"=w1623, "S4ACS_GUI in"=w1639) -> ("error out"=w1575:errorcluster, "S4ACS_GUI out"=w1576:refnum<class "S4GUI.lvclass">)  [unwired: 7 in]
        n821 = call "Write cfg file.vi"("error in (no error)"=w1575, "cfg file"="lastsaved.cfg", "S4ACS_GUI in"=w1576) -> ("error out"=w1578:errorcluster, "S4ACS_GUI out"=w1579:refnum<class "S4GUI.lvclass">)  [unwired: 7 in]
      }
      event "Set from Input ch3": Value Change {
        n822 = event-data() -> ()  [unwired: 1 in, 6 out]
        n823 = local read "Input Cluster"() -> (w1650:T5)
        n824 = Unbundle By Name(w1650) -> ("Parameters"=w1649:T23)
        n825 = Unbundle By Name(w1649) -> ("Image \nInitial Line"=w1678:u16, "Image\nInitial Column"=w1677:u16, "Image\nFinal Line"=w1676:u16, "Image\nFInal Column"=w1675:u16, "Vertical\nBinning"=w1674:u16, "Horizontal\nBinning"=w1673:u16, "Pre-amplification\nGain"=w1672:u8, "CCD\nEM Gain"=w1671:u16, "Readout\nRate"=w1670:u8, "Shutter\nOpenning Time"=w1669:i32, "Shutter\nClosing Time"=w1668:i32, "Vertical\nShift Speed"=w1667:u8, "Read\nMode"=w1666:u8, "Vertical\nClock Voltage"=w1665:u8, "A/D \nChannel"=w1664:u32, "Shutter\nMode"=w1663:u16, "Shutter\nTTL"=w1662:u16, "Trigger\nMode"=w1661:u16, "Frame\nTransfer"=w1660:bool, "Acquisition\nMode"=w1659:u8, "CCD \nEM Mode"=w1658:u8)
        n826 = call-dynamic "Read AcquisitionC.vi"("error in (no error)"=w1707, "S4ACS_GUI in"=w1708) -> ("error out"=w1701:errorcluster, "Acquisition.lvclass"=w1705:refnum<class "Acquisition.lvclass">, "S4ACS_GUI out"=w1706:refnum<class "S4GUI.lvclass">)  [unwired: 7 in]
        n827 = call-dynamic "Read Channel.vi"("error in (no error)"=w1701, "Acquisition in"=w1705) -> ("error out"=w1700:errorcluster, "Channel.lvclass"=w1703:refnum<class "Channel.lvclass">, "Acquisition out"=w1704:refnum<class "Acquisition.lvclass">)  [unwired: 7 in]
        n828 = call-dynamic "Read Interface.vi"("error in (no error)"=w1700, "Channel in"=w1703) -> ("error out"=w1682:errorcluster, "Interface.lvclass"=w1683:refnum<class "Interface.lvclass">, "Channel out"=w1702:refnum<class "Channel.lvclass">)  [unwired: 7 in]
        n829 = call-dynamic "Get CCD_Config.vi"("error in (no error)"=w1682, "Interface in"=w1683) -> ("error out"=w1679:errorcluster, "output cluster"=w1681:T24, "Interface out"=w1680:refnum<class "Interface.lvclass">)  [unwired: 7 in]
        n830 = Bundle By Name(cluster=w1681, "INITIAL_LINE"=w1678, "INITIAL_COLUMN"=w1677, "FINAL_LINE"=w1676, "FINAL_COLUMN"=w1675, "VBIN"=w1674, "HBIN"=w1673, "PREAMP"=w1672, "EM_GAIN"=w1671, "READOUT_RATE"=w1670, "SHUTTER_OPENING_TIME"=w1669, "SHUTTER_CLOSING_TIME"=w1668, "VERTICAL_SHIFT_SPEED"=w1667, "READ_MODE"=w1666, "VERTICAL_CLOCK_VOLTAGE"=w1665, "AD_CHANNEL"=w1664, "SHUTTER_MODE"=w1663, "SHUTTER_TTL"=w1662, "TRIGGER_MODE"=w1661, "FRAME_TRANSFER"=w1660, "ACQUISITION_MODE"=w1659, "EM_MODE"=w1658) -> (w1648:T24)
        n831 = call-dynamic "Set CCD_Config.vi"("error in (no error)"=w1679, "input cluster"=w1648, "Interface in"=w1680) -> ("error out"=w1686:errorcluster, "Interface out"=w1687:refnum<class "Interface.lvclass">)  [unwired: 7 in]
        n832 = Flatten To String(anything=w1648, error in (no error)=w1686) -> (data string=w1689:string, error out=w1688:errorcluster)  [unwired: 2 in, 1 out]
        n833 = call "Write flatted cluster.vi"("error in (no error)"=w1688, "flatted cluster"=w1689, "Interface in"=w1687) -> ("error out"=w1685:errorcluster, "Interface out"=w1684:refnum<class "Interface.lvclass">)  [unwired: 7 in]
        n834 = call-dynamic "Write Interface.vi"("error in (no error)"=w1685, "Interface.lvclass"=w1684, "Channel in"=w1702) -> ("error out"=w1653:errorcluster, "Channel out"=w1656:refnum<class "Channel.lvclass">)  [unwired: 7 in]
        n835 = call "Write section_name.vi"("error in (no error)"=w1653, "section_name"="CCD_ACS3", "Channel in"=w1656) -> ("error out"=w1652:errorcluster, "Channel out"=w1655:refnum<class "Channel.lvclass">)  [unwired: 7 in]
        n836 = call-dynamic "save config.vi"("error in (no error)"=w1652, "file config"="lastsaved.cfg", "Channel in"=w1655) -> ("error out"=w1651:errorcluster, "Channel out"=w1654:refnum<class "Channel.lvclass">)  [unwired: 7 in]
        n837 = call-dynamic "Read State Machine.vi"("error in (no error)"=w1651, "Device in"=w1654) -> ("error out"=w1696:errorcluster, "State Machine.lvclass"=w1698:refnum<class "State Machine.lvclass">, "Device out"=w1699:refnum<class "Channel.lvclass">)  [unwired: 7 in]
        n838 = call-dynamic "Write State.vi"("error in (no error)"=w1696, "State"=60, "State Machine in"=w1698) -> ("error out"=w1695:errorcluster, "State Machine out"=w1697:refnum<class "State Machine.lvclass">)  [unwired: 7 in]
        n839 = call-dynamic "Write State Machine.vi"("error in (no error)"=w1695, "State Machine.lvclass"=w1697, "Device in"=w1699) -> ("error out"=w1692:errorcluster, "Device out"=w1693:refnum<class "Channel.lvclass">)  [unwired: 7 in]
        n840 = call-dynamic "Write Channel.vi"("error in (no error)"=w1692, "Channel.lvclass"=w1693, "Acquisition in"=w1704) -> ("error out"=w1691:errorcluster, "Acquisition out"=w1690:refnum<class "Acquisition.lvclass">)  [unwired: 7 in]
        n841 = call-dynamic "Write AcquisitionC.vi"("error in (no error)"=w1691, "Acquisition.lvclass"=w1690, "S4ACS_GUI in"=w1706) -> ("error out"=w1642:errorcluster, "S4ACS_GUI out"=w1643:refnum<class "S4GUI.lvclass">)  [unwired: 7 in]
        n842 = call "Write cfg file.vi"("error in (no error)"=w1642, "cfg file"="lastsaved.cfg", "S4ACS_GUI in"=w1643) -> ("error out"=w1645:errorcluster, "S4ACS_GUI out"=w1646:refnum<class "S4GUI.lvclass">)  [unwired: 7 in]
      }
      event "Set from Input ch4": Value Change {
        n843 = event-data() -> ()  [unwired: 1 in, 6 out]
        n844 = local read "Input Cluster"() -> (w1717:T5)
        n845 = Unbundle By Name(w1717) -> ("Parameters"=w1716:T23)
        n846 = Unbundle By Name(w1716) -> ("Image \nInitial Line"=w1745:u16, "Image\nInitial Column"=w1744:u16, "Image\nFinal Line"=w1743:u16, "Image\nFInal Column"=w1742:u16, "Vertical\nBinning"=w1741:u16, "Horizontal\nBinning"=w1740:u16, "Pre-amplification\nGain"=w1739:u8, "CCD\nEM Gain"=w1738:u16, "Readout\nRate"=w1737:u8, "Shutter\nOpenning Time"=w1736:i32, "Shutter\nClosing Time"=w1735:i32, "Vertical\nShift Speed"=w1734:u8, "Read\nMode"=w1733:u8, "Vertical\nClock Voltage"=w1732:u8, "A/D \nChannel"=w1731:u32, "Shutter\nMode"=w1730:u16, "Shutter\nTTL"=w1729:u16, "Trigger\nMode"=w1728:u16, "Frame\nTransfer"=w1727:bool, "Acquisition\nMode"=w1726:u8, "CCD \nEM Mode"=w1725:u8)
        n847 = call-dynamic "Read AcquisitionD.vi"("error in (no error)"=w1774, "S4ACS_GUI in"=w1775) -> ("error out"=w1768:errorcluster, "Acquisition.lvclass"=w1772:refnum<class "Acquisition.lvclass">, "S4ACS_GUI out"=w1773:refnum<class "S4GUI.lvclass">)  [unwired: 7 in]
        n848 = call-dynamic "Read Channel.vi"("error in (no error)"=w1768, "Acquisition in"=w1772) -> ("error out"=w1767:errorcluster, "Channel.lvclass"=w1770:refnum<class "Channel.lvclass">, "Acquisition out"=w1771:refnum<class "Acquisition.lvclass">)  [unwired: 7 in]
        n849 = call-dynamic "Read Interface.vi"("error in (no error)"=w1767, "Channel in"=w1770) -> ("error out"=w1749:errorcluster, "Interface.lvclass"=w1750:refnum<class "Interface.lvclass">, "Channel out"=w1769:refnum<class "Channel.lvclass">)  [unwired: 7 in]
        n850 = call-dynamic "Get CCD_Config.vi"("error in (no error)"=w1749, "Interface in"=w1750) -> ("error out"=w1746:errorcluster, "output cluster"=w1748:T24, "Interface out"=w1747:refnum<class "Interface.lvclass">)  [unwired: 7 in]
        n851 = Bundle By Name(cluster=w1748, "INITIAL_LINE"=w1745, "INITIAL_COLUMN"=w1744, "FINAL_LINE"=w1743, "FINAL_COLUMN"=w1742, "VBIN"=w1741, "HBIN"=w1740, "PREAMP"=w1739, "EM_GAIN"=w1738, "READOUT_RATE"=w1737, "SHUTTER_OPENING_TIME"=w1736, "SHUTTER_CLOSING_TIME"=w1735, "VERTICAL_SHIFT_SPEED"=w1734, "READ_MODE"=w1733, "VERTICAL_CLOCK_VOLTAGE"=w1732, "AD_CHANNEL"=w1731, "SHUTTER_MODE"=w1730, "SHUTTER_TTL"=w1729, "TRIGGER_MODE"=w1728, "FRAME_TRANSFER"=w1727, "ACQUISITION_MODE"=w1726, "EM_MODE"=w1725) -> (w1715:T24)
        n852 = call-dynamic "Set CCD_Config.vi"("error in (no error)"=w1746, "input cluster"=w1715, "Interface in"=w1747) -> ("error out"=w1753:errorcluster, "Interface out"=w1754:refnum<class "Interface.lvclass">)  [unwired: 7 in]
        n853 = Flatten To String(anything=w1715, error in (no error)=w1753) -> (data string=w1756:string, error out=w1755:errorcluster)  [unwired: 2 in, 1 out]
        n854 = call "Write flatted cluster.vi"("error in (no error)"=w1755, "flatted cluster"=w1756, "Interface in"=w1754) -> ("error out"=w1752:errorcluster, "Interface out"=w1751:refnum<class "Interface.lvclass">)  [unwired: 7 in]
        n855 = call-dynamic "Write Interface.vi"("error in (no error)"=w1752, "Interface.lvclass"=w1751, "Channel in"=w1769) -> ("error out"=w1720:errorcluster, "Channel out"=w1723:refnum<class "Channel.lvclass">)  [unwired: 7 in]
        n856 = call "Write section_name.vi"("error in (no error)"=w1720, "section_name"="CCD_ACS4", "Channel in"=w1723) -> ("error out"=w1719:errorcluster, "Channel out"=w1722:refnum<class "Channel.lvclass">)  [unwired: 7 in]
        n857 = call-dynamic "save config.vi"("error in (no error)"=w1719, "file config"="lastsaved.cfg", "Channel in"=w1722) -> ("error out"=w1718:errorcluster, "Channel out"=w1721:refnum<class "Channel.lvclass">)  [unwired: 7 in]
        n858 = call-dynamic "Read State Machine.vi"("error in (no error)"=w1718, "Device in"=w1721) -> ("error out"=w1763:errorcluster, "State Machine.lvclass"=w1765:refnum<class "State Machine.lvclass">, "Device out"=w1766:refnum<class "Channel.lvclass">)  [unwired: 7 in]
        n859 = call-dynamic "Write State.vi"("error in (no error)"=w1763, "State"=60, "State Machine in"=w1765) -> ("error out"=w1762:errorcluster, "State Machine out"=w1764:refnum<class "State Machine.lvclass">)  [unwired: 7 in]
        n860 = call-dynamic "Write State Machine.vi"("error in (no error)"=w1762, "State Machine.lvclass"=w1764, "Device in"=w1766) -> ("error out"=w1759:errorcluster, "Device out"=w1760:refnum<class "Channel.lvclass">)  [unwired: 7 in]
        n861 = call-dynamic "Write Channel.vi"("error in (no error)"=w1759, "Channel.lvclass"=w1760, "Acquisition in"=w1771) -> ("error out"=w1758:errorcluster, "Acquisition out"=w1757:refnum<class "Acquisition.lvclass">)  [unwired: 7 in]
        n862 = call-dynamic "Write AcquisitionD.vi"("error in (no error)"=w1758, "Acquisition.lvclass"=w1757, "S4ACS_GUI in"=w1773) -> ("error out"=w1709:errorcluster, "S4ACS_GUI out"=w1710:refnum<class "S4GUI.lvclass">)  [unwired: 7 in]
        n863 = call "Write cfg file.vi"("error in (no error)"=w1709, "cfg file"="lastsaved.cfg", "S4ACS_GUI in"=w1710) -> ("error out"=w1712:errorcluster, "S4ACS_GUI out"=w1713:refnum<class "S4GUI.lvclass">)  [unwired: 7 in]
      }
      event "Restore Default ch1": Value Change {
        n864 = event-data() -> ()  [unwired: 1 in, 6 out]
        n865 = call-dynamic "Read AcquisitionA.vi"("error in (no error)"=w1806, "S4ACS_GUI in"=w1807) -> ("error out"=w1802:errorcluster, "Acquisition.lvclass"=w1804:refnum<class "Acquisition.lvclass">, "S4ACS_GUI out"=w1805:refnum<class "S4GUI.lvclass">)  [unwired: 7 in]
        n866 = call-dynamic "Read Channel.vi"("error in (no error)"=w1802, "Acquisition in"=w1804) -> ("error out"=w1789:errorcluster, "Channel.lvclass"=w1791:refnum<class "Channel.lvclass">, "Acquisition out"=w1803:refnum<class "Acquisition.lvclass">)  [unwired: 7 in]
        n867 = call "Write section_name.vi"("error in (no error)"=w1789, "section_name"="CCD_ACS1", "Channel in"=w1791) -> ("error out"=w1788:errorcluster, "Channel out"=w1790:refnum<class "Channel.lvclass">)  [unwired: 7 in]
        n868 = call-dynamic "load config.vi"("error in (no error)"=w1788, "cfg file name"="default.cfg", "Channel in"=w1790) -> ("error out"=w1786:errorcluster, "Channel out"=w1787:refnum<class "Channel.lvclass">)  [unwired: 7 in]
        n869 = call-dynamic "Read State Machine.vi"("error in (no error)"=w1786, "Device in"=w1787) -> ("error out"=w1798:errorcluster, "State Machine.lvclass"=w1800:refnum<class "State Machine.lvclass">, "Device out"=w1801:refnum<class "Channel.lvclass">)  [unwired: 7 in]
        n870 = call-dynamic "Write State.vi"("error in (no error)"=w1798, "State"=60, "State Machine in"=w1800) -> ("error out"=w1797:errorcluster, "State Machine out"=w1799:refnum<class "State Machine.lvclass">)  [unwired: 7 in]
